vi "Display queue status.vi"(6 "action":enum16{"Init", "Get", "Set"}(ring)=enum."Set", 7 "error in":errorcluster, 9 "enqueue channel in":enum16{"1", "2"}(ring)=enum."2", 10 "dequeue channel in":enum16{"1", "2"}(ring)=enum."2") -> (0 "error out":errorcluster, 2 "dequeue channel out":enum16{"1", "2"}(ring), 3 "enqueue channel out":enum16{"1", "2"}(ring))   [LabVIEW 2018]
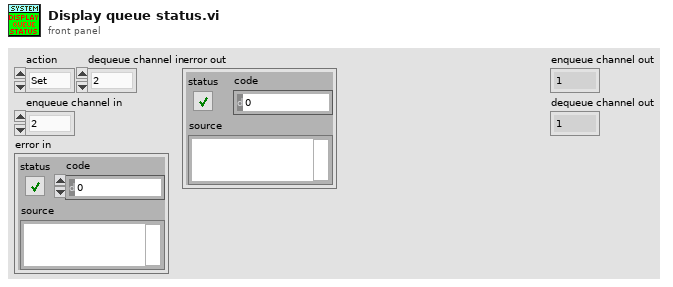
[diagram p1: front panel]
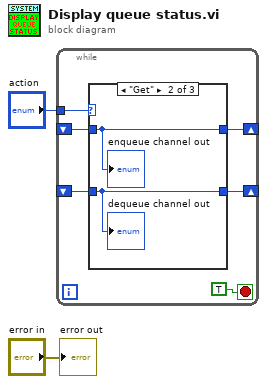
[diagram p0: block diagram]
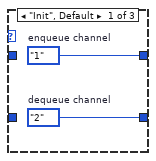
[diagram p2: hidden frame]
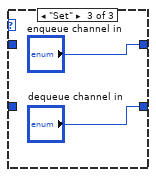
[diagram p3: hidden frame]
diagram:
  n1 = while {
    tunnel: "action" -> [w7]
    shift-right: [w6] -> _
    shift-left: _ -> [w4]
    shift-right: [w5] -> _
    shift-left: _ -> [w3]
    stop <- TRUE stop-if-true
    n2 = case shown="\"Get\"" w7 {
      tunnel: [w10 w12 "enqueue channel in"] -> w6
      tunnel: [w9 w11 "dequeue channel in"] -> w5
      tunnel: w4 -> [_ w12 _]
      tunnel: w3 -> [_ w11 _]
      frame "Init", Default {
        w9 = enum16{"1", "2"}."2"  # dequeue channel
        w10 = enum16{"1", "2"}."1"  # enqueue channel
      }
      frame "Get" {
        "enqueue channel out" <- w12
        "dequeue channel out" <- w11
      }
      frame "Set" {
      }
    }
  }
  "error out" <- "error in"
